vi "手动加载电流.vi"(2 "电源台数":dbl, 5 "停止":bool, 7 "延迟时间":dbl, 8 "error in (no error)":errorcluster, 9 "电流(A)":dbl, 10 "循环次数":i32, 11 "VISA resource name out":refnum<visa-resource-name>) -> (0 "error out":errorcluster, 3 "VISA resource name out 2":refnum<visa-resource-name>, 4 "表格控件":string[][](table), 6 "已循环次数":i32)   [LabVIEW 2021]
uses:
  <instrlib>/TDK-Lambda G Series/TDK-Lambda G Series.lvlib
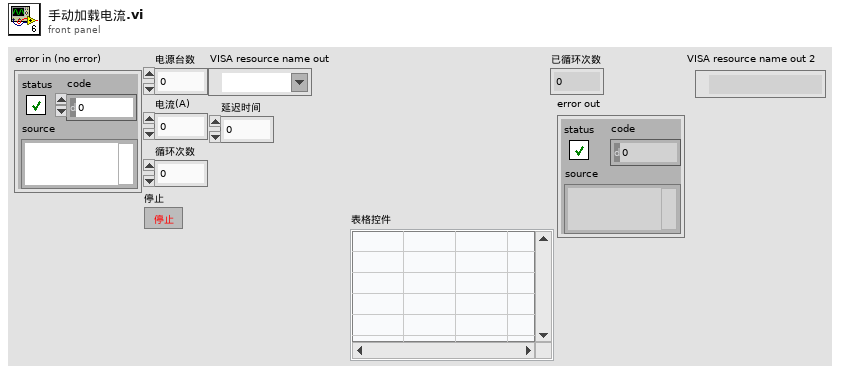
[diagram p1: front panel]
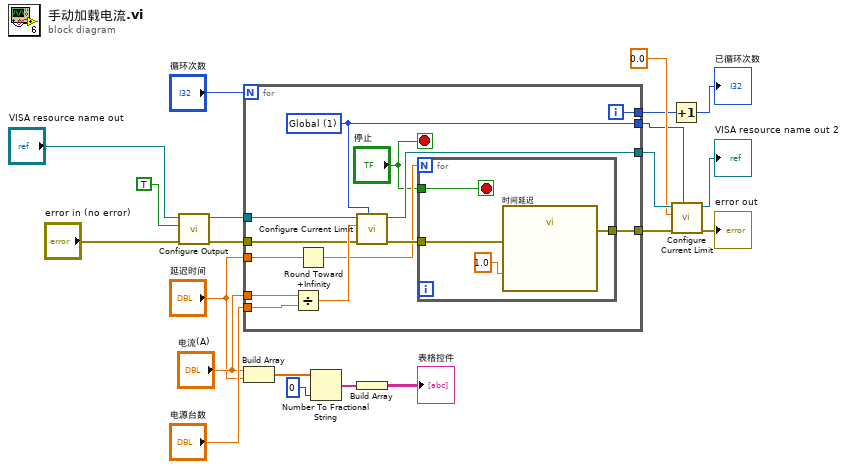
[diagram p0: block diagram]
diagram:
  n1 = call <instrlib>:"Configure Output.vi"("error in (no error)"="error in (no error)", "Enable Output (False)"=TRUE, "VISA resource name"="VISA resource name out") -> ("error out"=w2:errorcluster, "VISA resource name out"=w4:refnum<visa-resource-name>)  [unwired: 7 in]
  n2 = for {
    N: "循环次数" -> [_]
    tunnel: w4 -> [w34]
    tunnel: [w23] -> w21
    tunnel: [w32] -> w20
    tunnel: [w31] -> w18
    tunnel: [w29] -> w17
    tunnel: "电流(A)" -> [w28]
    tunnel: "延迟时间" -> [w27]
    tunnel: w2 -> [w25]
    tunnel: "电源台数" -> [w24]
    i -> [w29]
    stop <- "停止" stop-if-true
    w31 = u16 1 items=["Single", "Global"] ("Globalize (0: Single)")
    n3 = Divide(x=w28, y=w24) -> (x/y=w30:dbl)
    n4 = Round Toward +Infinity(x=w27) -> (ceil(x): smallest int >= x=w26:dbl)
    n5 = call <instrlib>:"Configure Current Limit.vi"("Globalize (0: Single)"=w31, "error in (no error)"=w25, "Current Limit (0A)"=w30, "VISA resource name"=w34) -> ("error out"=w33:errorcluster, "VISA resource name out"=w32:refnum<visa-resource-name>)  [unwired: 6 in]
    n6 = for {
      N: w26 -> [_]
      tunnel: w33 -> [w38]
      tunnel: [w37] -> w23
      tunnel: "停止" -> [w35]
      stop <- w35 stop-if-true
      n7 = call "时间延迟"("error in (no error)"=w38, "Delay Time (s)"=1.0) -> ("error out"=w37:errorcluster)  [unwired: 9 in]
    }
  }
  n8 = Build Array("电流(A)", "延迟时间") -> (w16:dbl[])
  n9 = Number To Fractional String(number=w16, precision (6)=i16 0 ("精度(6)")) -> (F-format string=w15:string[])  [unwired: 2 in]
  n10 = Build Array(w15) -> (→"表格控件":string[][])
  n11 = Increment(x=w17) -> (x+1=→"已循环次数":i32)
  n12 = call <instrlib>:"Configure Current Limit.vi"("Globalize (0: Single)"=w18, "error in (no error)"=w21, "Current Limit (0A)"=0.0, "VISA resource name"=w20) -> ("error out"=→"error out":errorcluster, "VISA resource name out"=→"VISA resource name out 2":refnum<visa-resource-name>)  [unwired: 6 in]
